vi "check_if_configuration_exists.vi"(8 "error in (no error)":errorcluster, 11 "number of strips":i32=4) -> (0 "error out":errorcluster)   [LabVIEW 2010]
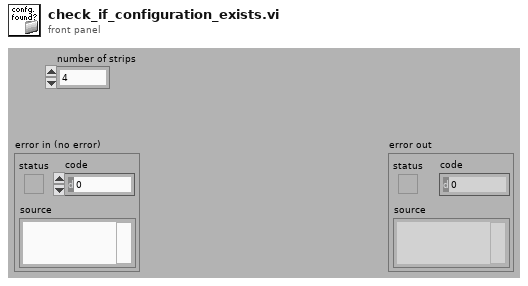
[diagram p1: front panel]
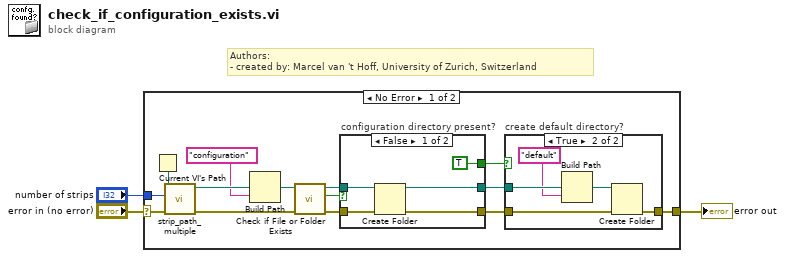
[diagram p0: block diagram]
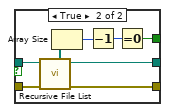
[diagram p3: hidden frame]
diagram:
  # "Authors: \n- created by: Marcel van 't Hoff, University of Zurich, Switzerland"
  n1 = case shown="No Error" "error in (no error)" {
    selector: "error in (no error)" -> [w17 w37]
    tunnel: [w7 w37] -> w2
    tunnel: "number of strips" -> [w4 _]
    frame No Error {
      n2 = Current VI's Path() -> (path=w16:path)
      n3 = call "strip_path_multiple.vi"("error in (no error)"=w17, "number of strips"=w4, "path in"=w16) -> ("error out"=w12:errorcluster, "path out"=w15:path)  [unwired: 7 in]
      n4 = Build Path(base path=w15, name or relative path="configuration") -> (appended path=w13:path)
      n5 = call <vilib>:"Check if File or Folder Exists.vi"("error in (no error)"=w12, "path"=w13) -> ("error out"=w9:errorcluster, "file or folder exists?"=w11:bool, "dup path"=w10:path)  [unwired: 7 in]
      n6 = case "configuration directory present?" shown="False" w11 {
        tunnel: w10 -> [w28 w36]
        tunnel: w9 -> [w26 w35]
        tunnel: [TRUE w31] -> w8
        tunnel: [w25 w30] -> w6
        tunnel: [w27 w29] -> w5
        frame False {
          n7 = Create Folder(path (use dialog)=w28, error in=w26) -> (created path=w27:path, error out=w25:errorcluster)  [unwired: 1 in, 1 out]
        }
        frame True {
          n8 = call <vilib>:"Recursive File List.vi"("error in (no error)"=w35, "Folder Path"=w36) -> ("error out"=w30:errorcluster, "dup Folder Path"=w29:path, "All Folders"=w34:path[])  [unwired: 5 in, 2 out]
          n9 = Array Size(array=w34) -> (size(s)=w33:i32)
          n10 = Decrement(x=w33) -> (x-1=w32:i32)
          n11 = Equal To 0?(x=w32) -> (x = 0?=w31:bool)
        }
      }
      n12 = case "create default directory?" shown="True" w8 {
        tunnel: [w18 w22] -> w7
        tunnel: w6 -> [w18 w23]
        tunnel: w5 -> [_ w21]
        frame False {
        }
        frame True {
          n13 = Build Path(base path=w21, name or relative path="default") -> (appended path=w20:path)
          n14 = Create Folder(path (use dialog)=w20, error in=w23) -> (error out=w22:errorcluster)  [unwired: 1 in, 2 out]
        }
      }
    }
    frame Error {
    }
  }
  "error out" <- w2
